vi "IMAQ-GetRMSContrast.vi"(1 "Intensity 2D Array":dbl[][](array[numeric])) -> (0 "RMS Contrast":dbl)   [LabVIEW 2010]
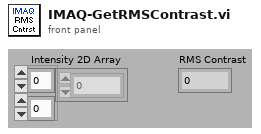
[diagram p1: front panel]
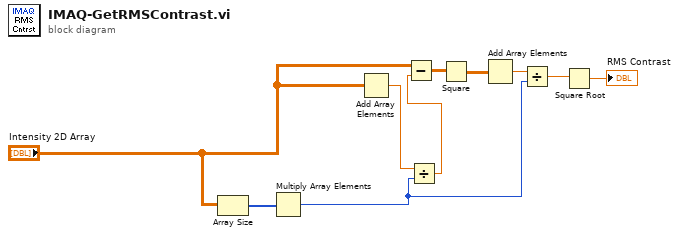
[diagram p0: block diagram]
diagram:
  n1 = Array Size(array="Intensity 2D Array") -> (size(s)=w3:i32[])
  n2 = Multiply Array Elements(1:w3) -> (0:w1:i32)
  n3 = Add Array Elements(numeric array="Intensity 2D Array") -> (sum=w5:dbl)
  n4 = Divide(x=w5, y=w1) -> (x/y=w4:dbl)
  n5 = Subtract(x="Intensity 2D Array", y=w4) -> (x-y=w6:dbl[][])
  n6 = Square(x=w6) -> (x^2=w7:dbl[][])
  n7 = Add Array Elements(numeric array=w7) -> (sum=w8:dbl)
  n8 = Divide(x=w8, y=w1) -> (x/y=w9:dbl)
  n9 = Square Root(x=w9) -> (sqrt(x)=→"RMS Contrast":dbl)
